vi "Path Loss Compensation - NF.vi"(8 "error in (no error)":errorcluster, 10 "Path Losses":T1={"DUT Input Loss"={"Compensation Enabled"=0, "Temperation (K)"=0.0, "S2P Path"=path "C:/Users/ies-pg-8881/Desktop/KB/CMT/PS_ATT6dB_26.5GHz.csv", "Orientation"=enum."Port1 Towards DUT"}, "DUT Output Loss"={"Compensation Enabled"=0, "Temperation (K)"=0.0, "S2P Path"=path "C:/Users/ies-pg-8881/Desktop/KB/CMT/PS_ATT6dB_26.5GHz.csv", "Orientation"=enum."Port1 Towards DUT"}, "Calibration Loss"={"Compensation Enabled"=0, "Temperation (K)"=0.0, "S2P Path"=path "C:/Users/ies-pg-8881/Desktop/KB/CMT/PS_ATT6dB_26.5GHz.csv", "Orientation"=enum."Port1 Towards DUT"}, "Noise Source Loss"={"Compensation Enabled"=0, "Temperation (K)"=0.0, "S2P Path"=path "C:/Users/ies-pg-8881/Desktop/KB/CMT/PS_ATT6dB_26.5GHz.csv", "Orientation"=enum."Port1 Towards DUT"}} {"Noise Source Loss"."Compensation Enabled" items=["False", "True"]; "Noise Source Loss"."Temperation (K)" format="%.2g"; "Calibration Loss"."Compensation Enabled" items=["False", "True"]; "Calibration Loss"."Temperation (K)" format="%.2g"; "DUT Output Loss"."Compensation Enabled" items=["False", "True"]; "DUT Output Loss"."Temperation (K)" format="%.2g"; "DUT Input Loss"."Compensation Enabled" items=["False", "True"]; "DUT Input Loss"."Temperation (K)" format="%.2g"}, 11 "RFmx Session in":refnum<k21>) -> (0 "error out":errorcluster, 3 "RFmx Session out":refnum<k21>)   [LabVIEW 2023]
uses:
  Controls/Path Loss Settings Cluster.ctl
  Controls/Path Loss Settings.ctl
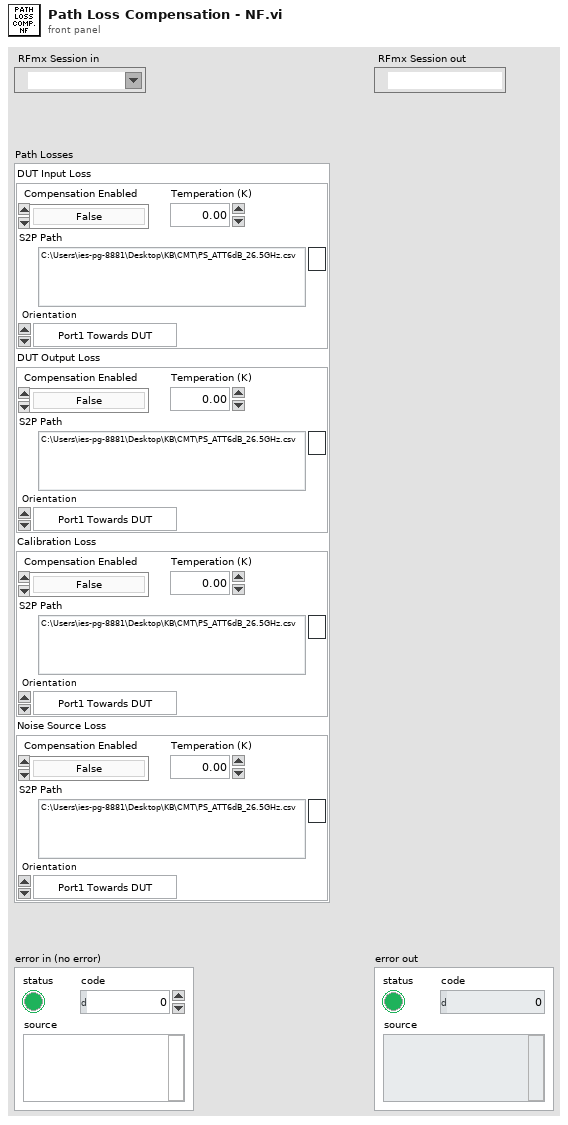
[diagram p1: front panel]
types:
  T1 = typedef "Path Loss Settings Cluster.ctl" = cluster{"DUT Input Loss":T2, "DUT Output Loss":T2, "Calibration Loss":T2, "Noise Source Loss":T2}
  T2 = typedef "Path Loss Settings.ctl" = cluster{"Compensation Enabled":i32, "Temperation (K)":dbl, "S2P Path":path, "Orientation":enum32{"Port1 Towards DUT", "Port2 Towards DUT"}}
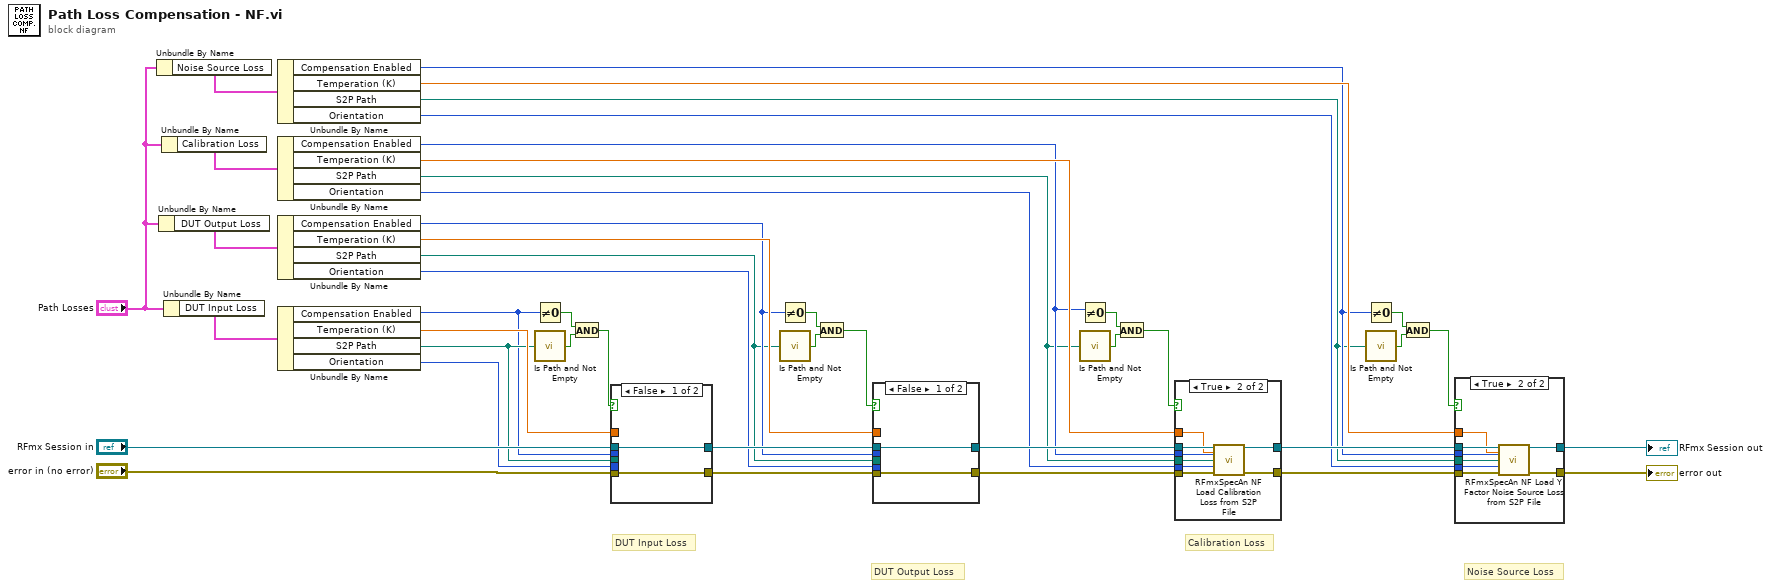
[diagram p0: block diagram]
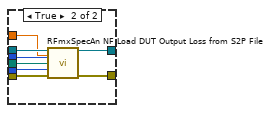
[diagram p4: hidden frame]
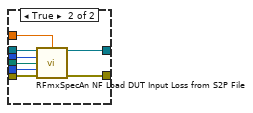
[diagram p5: hidden frame]
diagram:
  # "Noise Source Loss"
  # "Calibration Loss"
  # "DUT Output Loss"
  # "DUT Input Loss"
  n1 = Unbundle By Name("Path Losses") -> ("Noise Source Loss"=w40:T2)
  n2 = Unbundle By Name("Path Losses") -> ("DUT Output Loss"=w41:T2)
  n3 = Unbundle By Name("Path Losses") -> ("Calibration Loss"=w42:T2)
  n4 = Unbundle By Name("Path Losses") -> ("DUT Input Loss"=w43:T2)
  n5 = Unbundle By Name(w40) -> ("Compensation Enabled"=w2:i32, "Temperation (K)"=w28:dbl, "S2P Path"=w1:path, "Orientation"=w21:enum32{"Port1 Towards DUT", "Port2 Towards DUT"})
  n6 = Unbundle By Name(w42) -> ("Compensation Enabled"=w7:i32, "Temperation (K)"=w25:dbl, "S2P Path"=w6:path, "Orientation"=w22:enum32{"Port1 Towards DUT", "Port2 Towards DUT"})
  n7 = Unbundle By Name(w41) -> ("Compensation Enabled"=w12:i32, "Temperation (K)"=w27:dbl, "S2P Path"=w11:path, "Orientation"=w23:enum32{"Port1 Towards DUT", "Port2 Towards DUT"})
  n8 = Unbundle By Name(w43) -> ("Compensation Enabled"=w17:i32, "Temperation (K)"=w26:dbl, "S2P Path"=w20:path, "Orientation"=w24:enum32{"Port1 Towards DUT", "Port2 Towards DUT"})
  n9 = Not Equal To 0?(x=w17) -> (x != 0?=w16:bool)
  n10 = call <vilib>:"Is Path and Not Empty.vi"("path"=w20) -> ("Is Path and Not Empty?"=w18:bool)  [unwired: 4 in]
  n11 = And(x=w16, y=w18) -> (x .and. y?=w19:bool)
  n12 = case shown="False" w19 {
    tunnel: [w44 w53] -> w32
    tunnel: [w45 w52] -> w31
    tunnel: "error in (no error)" -> [w44 w51]
    tunnel: "RFmx Session in" -> [w45 w50]
    tunnel: w26 -> [_ w49]
    tunnel: w17 -> [_ w48]
    tunnel: w20 -> [_ w47]
    tunnel: w24 -> [_ w46]
    frame False {
    }
    frame True {
      n13 = call <vilib>:"RFmxSpecAn NF Load DUT Input Loss from S2P File.vi"("Instrument Handle In"=w50, "DUT Input Loss Temperature (K)"=w49, "DUT Input Loss Compensation Enabled"=w48, "DUT Input Loss S2P File Path"=w47, "DUT Input Loss S-Parameter Orientation"=w46, "error in (no error)"=w51) -> ("Instrument Handle Out"=w52:refnum<k21>, "error out"=w53:errorcluster)  [unwired: 8 in]
    }
  }
  n14 = Not Equal To 0?(x=w12) -> (x != 0?=w15:bool)
  n15 = call <vilib>:"Is Path and Not Empty.vi"("path"=w11) -> ("Is Path and Not Empty?"=w14:bool)  [unwired: 4 in]
  n16 = And(x=w15, y=w14) -> (x .and. y?=w13:bool)
  n17 = case shown="False" w13 {
    tunnel: [w54 w63] -> w34
    tunnel: [w55 w62] -> w33
    tunnel: w32 -> [w54 w61]
    tunnel: w31 -> [w55 w60]
    tunnel: w27 -> [_ w59]
    tunnel: w12 -> [_ w58]
    tunnel: w23 -> [_ w57]
    tunnel: w11 -> [_ w56]
    frame False {
    }
    frame True {
      n18 = call <vilib>:"RFmxSpecAn NF Load DUT Output Loss from S2P File.vi"("Instrument Handle In"=w60, "DUT Output Loss Temperature (K)"=w59, "DUT Output Loss Compensation Enabled"=w58, "DUT Output Loss S2P File Path"=w56, "DUT Output Loss S-Parameter Orientation"=w57, "error in (no error)"=w61) -> ("Instrument Handle Out"=w62:refnum<k21>, "error out"=w63:errorcluster)  [unwired: 8 in]
    }
  }
  n19 = Not Equal To 0?(x=w7) -> (x != 0?=w9:bool)
  n20 = call <vilib>:"Is Path and Not Empty.vi"("path"=w6) -> ("Is Path and Not Empty?"=w10:bool)  [unwired: 4 in]
  n21 = And(x=w9, y=w10) -> (x .and. y?=w8:bool)
  n22 = case shown="True" w8 {
    tunnel: [w64 w73] -> w36
    tunnel: [w65 w72] -> w35
    tunnel: w34 -> [w64 w71]
    tunnel: w33 -> [w65 w70]
    tunnel: w25 -> [_ w69]
    tunnel: w7 -> [_ w68]
    tunnel: w22 -> [_ w67]
    tunnel: w6 -> [_ w66]
    frame False {
    }
    frame True {
      n23 = call <vilib>:"RFmxSpecAn NF Load Calibration Loss from S2P File.vi"("Instrument Handle In"=w70, "Calibration Loss Temperature (K)"=w69, "Calibration Loss Compensation Enabled"=w68, "Calibration Loss S2P File Path"=w66, "Calibration Loss S-Parameter Orientation"=w67, "error in (no error)"=w71) -> ("Instrument Handle Out"=w72:refnum<k21>, "error out"=w73:errorcluster)  [unwired: 8 in]
    }
  }
  n24 = Not Equal To 0?(x=w2) -> (x != 0?=w5:bool)
  n25 = call <vilib>:"Is Path and Not Empty.vi"("path"=w1) -> ("Is Path and Not Empty?"=w4:bool)  [unwired: 4 in]
  n26 = And(x=w5, y=w4) -> (x .and. y?=w3:bool)
  n27 = case shown="True" w3 {
    tunnel: [w74 w83] -> w39
    tunnel: [w75 w82] -> w38
    tunnel: w36 -> [w74 w81]
    tunnel: w35 -> [w75 w80]
    tunnel: w28 -> [_ w79]
    tunnel: w2 -> [_ w78]
    tunnel: w21 -> [_ w77]
    tunnel: w1 -> [_ w76]
    frame False {
    }
    frame True {
      n28 = call <vilib>:"RFmxSpecAn NF Load Y Factor Noise Source Loss from S2P File.vi"("Instrument Handle In"=w80, "Noise Source Loss Temperature (K)"=w79, "Noise Source Loss Compensation Enabled"=w78, "Noise Source Loss S2P File Path"=w76, "Noise Source Loss S-Parameter Orientation"=w77, "error in (no error)"=w81) -> ("Instrument Handle Out"=w82:refnum<k21>, "error out"=w83:errorcluster)  [unwired: 8 in]
    }
  }
  "error out" <- w39
  "RFmx Session out" <- w38
